vi "Decode Array Element Data.vi"(10 "Prepended Length":bool, 11 "Encoder Data Description":string) -> (3 "Array Data Element":T1)   [LabVIEW 2021, in "CIF_NI_CIPC.lvlib"]
uses:
  CIF_NI_CIPC.lvlib
  TypeDefs/Alignment.ctl
  <vilib>/CIF Foundation/CIF Utilities/DataTypes/Typedef/Endian.ctl
  <vilib>/CIF Foundation/CIF Utilities/DataTypes/DataTypes_CIF_U.lvlib
  TypeDefs/Data Struct Info.ctl
  TypeDefs/Data Struct Array Info.ctl
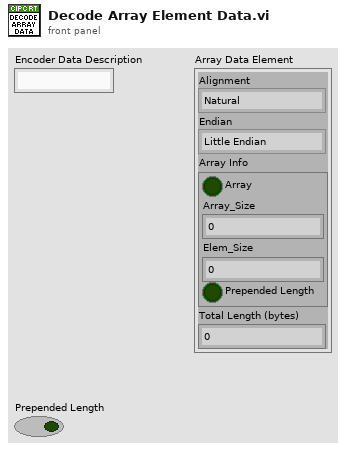
[diagram p1: front panel]
types:
  T1 = typedef "CIF_NI_CIPC.lvlib/Data Struct Info.ctl" = cluster{"Alignment":T2, "Endian":T3, "Array Info":T4, "Total Length (bytes)":i32}
  T2 = typedef "CIF_NI_CIPC.lvlib/Alignment.ctl" = enum16{"Natural", "Packed"}
  T3 = typedef "DataTypes_CIF_U.lvlib/Endian.ctl" = enum16{"Little Endian", "Big Endian"}
  T4 = typedef "CIF_NI_CIPC.lvlib/Data Struct Array Info.ctl" = cluster{"Array":bool, "Array_Size":i32, "Elem_Size":i32, "Prepended Length":bool}
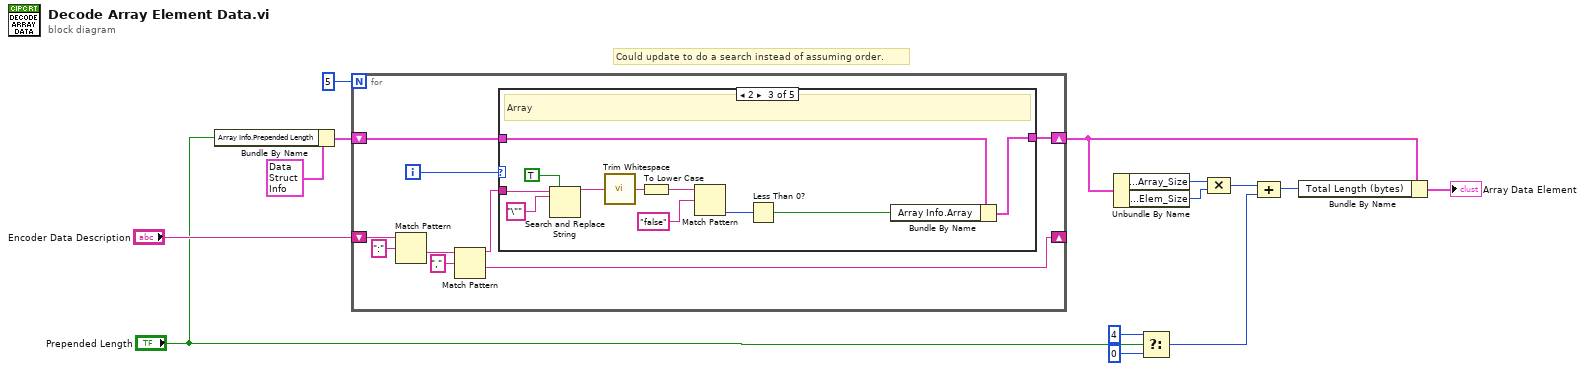
[diagram p0: block diagram]
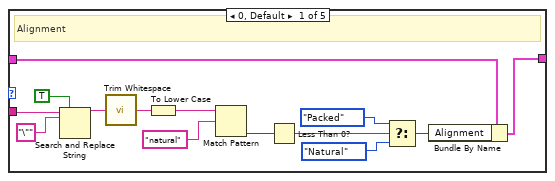
[diagram p2: hidden frame]
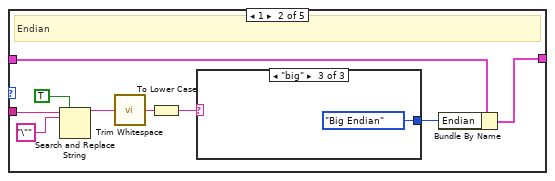
[diagram p3: hidden frame]
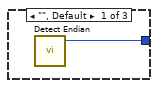
[diagram p4: hidden frame]
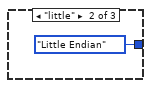
[diagram p5: hidden frame]
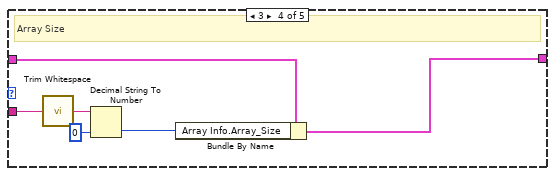
[diagram p6: hidden frame]
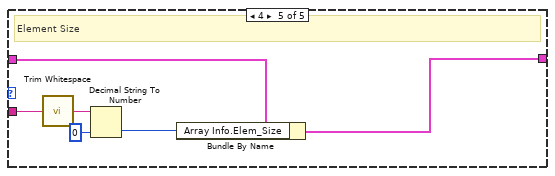
[diagram p7: hidden frame]
diagram:
  # "Could update to do a search instead of assuming order."
  n1 = Bundle By Name(cluster=T1 {"Alignment"=enum."Natural", "Endian"=enum."Little Endian", "Array Info"={"Array"=FALSE, "Array_Size"=0, "Elem_Size"=0, "Prepended Length"=FALSE}, "Total Length (bytes)"=0} ("Array Data Element"), "Array Info.Prepended Length"="Prepended Length") -> (w2:T1)
  n2 = for {
    N: 5 -> [_]
    shift-right: [w19] -> _
    shift-left: "Encoder Data Description" -> [w20]
    shift-right: [w15] -> w4
    shift-left: w2 -> [w17]
    i -> [w16]
    n3 = Match Pattern(string=w20, regular expression=":") -> (after substring=w22:string)  [unwired: 1 in, 3 out]
    n4 = Match Pattern(string=w22, regular expression=",") -> (before substring=w18:string, after substring=w19:string)  [unwired: 1 in, 2 out]
    n5 = case shown="2" w16 {
      tunnel: w18 -> [w37 w46 w60 w64 w71]
      tunnel: w17 -> [w33 w42 w56 w66 w67]
      tunnel: [w32 w41 w55 w65 w72] -> w15
      frame 0, Default {
        # "Alignment"
        n6 = Search and Replace String(replace all?=TRUE ("replace all? (F)"), input string=w37, search string="\"") -> (result string=w35:string)  [unwired: 5 in, 3 out]
        n7 = call <vilib>:"Trim Whitespace.vi"("string"=w35) -> ("trimmed string"=w31:string)  [unwired: 1 in]
        n8 = To Lower Case(string=w31) -> (all lower case string=w24:string)
        n9 = Match Pattern(string=w24, regular expression="natural") -> (offset past match=w30:i32)  [unwired: 1 in, 3 out]
        n10 = Less Than 0?(x=w30) -> (x < 0?=w28:bool)
        n11 = Select(t=Alignment."Packed", s=w28, f=Alignment."Natural" ("Alignment")) -> (s? t:f=w25:T2)
        n12 = Bundle By Name(cluster=w33, "Alignment"=w25) -> (w32:T1)
      }
      frame 1 {
        # "Endian"
        n13 = Search and Replace String(replace all?=TRUE ("replace all? (F)"), input string=w46, search string="\"") -> (result string=w44:string)  [unwired: 5 in, 3 out]
        n14 = call <vilib>:"Trim Whitespace.vi"("string"=w44) -> ("trimmed string"=w40:string)  [unwired: 1 in]
        n15 = To Lower Case(string=w40) -> (all lower case string=w39:string)
        n16 = case shown="\"big\"" w39 {
          tunnel: [w47 Endian."Little Endian" ("Endian") Endian."Big Endian" ("Endian")] -> w38
          frame "", Default {
            n17 = call <vilib>:"Detect Endian.vi"() -> ("Endian"=w47:T3)  [unwired: 5 in]
          }
          frame "little" {
          }
          frame "big" {
          }
        }
        n18 = Bundle By Name(cluster=w42, "Endian"=w38) -> (w41:T1)
      }
      frame 2 {
        # "Array"
        n19 = Search and Replace String(replace all?=TRUE ("replace all? (F)"), input string=w60, search string="\"") -> (result string=w58:string)  [unwired: 5 in, 3 out]
        n20 = call <vilib>:"Trim Whitespace.vi"("string"=w58) -> ("trimmed string"=w54:string)  [unwired: 1 in]
        n21 = To Lower Case(string=w54) -> (all lower case string=w51:string)
        n22 = Match Pattern(string=w51, regular expression="false") -> (offset past match=w53:i32)  [unwired: 1 in, 3 out]
        n23 = Less Than 0?(x=w53) -> (x < 0?=w50:bool)
        n24 = Bundle By Name(cluster=w56, "Array Info.Array"=w50) -> (w55:T1)
      }
      frame 3 {
        # "Array Size"
        n25 = call <vilib>:"Trim Whitespace.vi"("string"=w64) -> ("trimmed string"=w63:string)  [unwired: 1 in]
        n26 = Decimal String To Number(string=w63, default (0L)=0 ("default (0 I32)")) -> (number=w61:i32)  [unwired: 1 in, 1 out]
        n27 = Bundle By Name(cluster=w66, "Array Info.Array_Size"=w61) -> (w65:T1)
      }
      frame 4 {
        # "Element Size"
        n28 = call <vilib>:"Trim Whitespace.vi"("string"=w71) -> ("trimmed string"=w70:string)  [unwired: 1 in]
        n29 = Decimal String To Number(string=w70, default (0L)=0 ("default (0 I32)")) -> (number=w68:i32)  [unwired: 1 in, 1 out]
        n30 = Bundle By Name(cluster=w67, "Array Info.Elem_Size"=w68) -> (w72:T1)
      }
    }
  }
  n31 = Unbundle By Name(w4) -> ("Array Info.Array_Size"=w12:i32, "Array Info.Elem_Size"=w11:i32)
  n32 = Select(t=4, s="Prepended Length", f=0 ("Array Info.Elem_Size")) -> (s? t:f=w9:i32)
  n33 = Compound Arithmetic op=MULTIPLY(w12, w11) -> (w10:i32)
  n34 = Compound Arithmetic op=ADD(w10, w9) -> (w6:i32)
  n35 = Bundle By Name(cluster=w4, "Total Length (bytes)"=w6) -> (→"Array Data Element":T1)
